vi "Send M1M3 Summary State Event.vi"(8 "error in (no error)":errorcluster, 10 "logevent_SummaryState":T1, 11 "M1M3 Support Events in":refnum<class "M1M3 Support Events.lvclass">) -> (0 "error out":errorcluster, 3 "M1M3 Support Events out":refnum<class "M1M3 Support Events.lvclass">)   [LabVIEW 2016, in "M1M3 Support Events.lvclass"]
uses:
  M1M3 Support Events.lvclass
  SALLV_m1m3/DataTypes/logevent_SummaryState.ctl
  M1M3 Support Events.lvclass/M1M3 Support Events.ctl
  SALLV_m1m3/SALLV_m1m3.lvlib
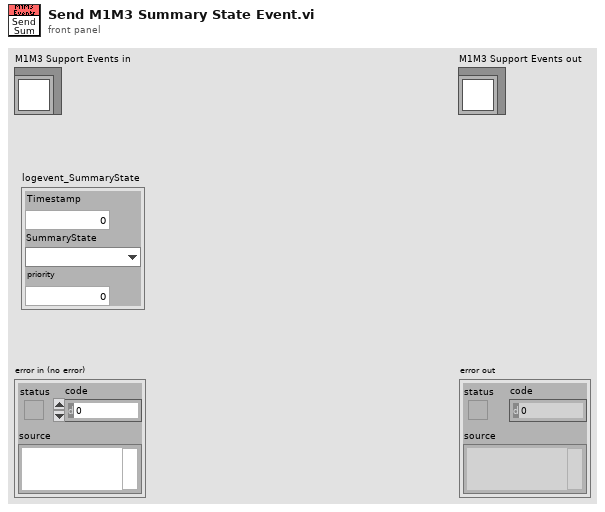
[diagram p1: front panel]
types:
  T1 = typedef "SALLV_m1m3.lvlib/logevent_SummaryState.ctl" = cluster{"Timestamp":dbl, "SummaryState":enum16{"", "SummaryState_SummaryStates_DisabledState", "SummaryState_SummaryStates_EnabledState", "SummaryState_SummaryStates_FaultState", "SummaryState_SummaryStates_OfflineState", "SummaryState_SummaryStates_StandbyState"}, "priority":i32}
  T2 = typedef "M1M3SupportEUI_TypeDefs.lvlib/M1M3 Support Events.ctl" = cluster{"Inclinometer  Data":refnum<user-event>, "IMS Data":refnum<user-event>, "SAL Connected":refnum<user-event>, "Accelerometer Data":refnum<user-event>, "OuterLoop Data":refnum<user-event>, "ErrorCode Event":refnum<user-event>, "InterlockStatus Event":refnum<user-event>, "InterlockWarning Event":refnum<user-event>, "Gyro Data":refnum<user-event>, "HP Actuator Info Event":refnum<user-event>, " FA Info Event":refnum<user-event>, "HP Monitor Info Event":refnum<user-event>, "FA Data":refnum<user-event>, "HP Actuator data":refnum<user-event>, "HP Monitor data":refnum<user-event>, "Air Supply Status Event":refnum<user-event>, "Air Supply Warning Event":refnum<user-event>, "Power Data":refnum<user-event>, "PID Data":refnum<user-event>, "PID Info Event":refnum<user-event>, "Power Status Event":refnum<user-event>, "Power Supply Status Event":refnum<user-event>, "Power Warning Event":refnum<user-event>, "Summary State Event":refnum<user-event>, "Detailed State Event":refnum<user-event>, "FA Force Warning Event":refnum<user-event>, "FA Warning Event":refnum<user-event>, "FA State Event":refnum<user-event>, "Applied AberrationForces Event":refnum<user-event>, "Applied Acceleration Forcces Event":refnum<user-event>, "Applied Azimuth Forces Event":refnum<user-event>, "Applied Active Optic Forces Event":refnum<user-event>, "Applied Balance Forces Event":refnum<user-event>, "Applied Cylinder Forces Event":refnum<user-event>, "Applied Elevation Forces Event":refnum<user-event>, "Applied Forces Event":refnum<user-event>, "Applied Offset Forces Event":refnum<user-event>, "Applied Static Forces Event":refnum<user-event>, "Applied Thermal Forces Event":refnum<user-event>, "Applied Velocity Forces Event":refnum<user-event>, "Rejected Aberration Force Event":refnum<user-event>, "Rejected Acceleration Forces Event":refnum<user-event>, "Rejected Active Optic Forces Event":refnum<user-event>, "Rejected Azimuth Forces Event":refnum<user-event>, "Rejected Balance Forces Event":refnum<user-event>, "Rejected Cylinder Forces Event":refnum<user-event>, "Rejected Elevation Forces Event":refnum<user-event>, "Rejected Forces Event":refnum<user-event>, "Rejected Offset Forces Event":refnum<user-event>, "Rejected Static Forces Event":refnum<user-event>, "Rejected Thermal Forces Event":refnum<user-event>, "Rejected Velocity Forces Event":refnum<user-event>, "Command Rejection Event":refnum<user-event>, "Setting Verions Event":refnum<user-event>, "Settings Applied Event":refnum<user-event>}
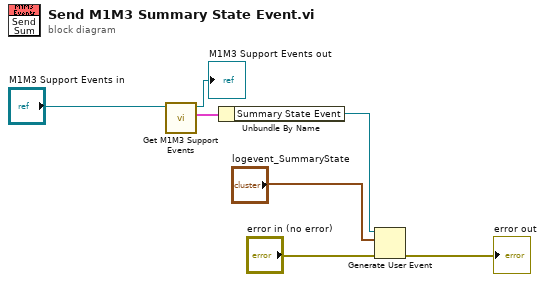
[diagram p0: block diagram]
diagram:
  n1 = call "Get M1M3 Support Events.vi"("M1M3 Support Events in"="M1M3 Support Events in") -> ("M1M3 Support Events"=w7:T2, "M1M3 Support Events out"=→"M1M3 Support Events out":refnum<class "M1M3 Support Events.lvclass">)  [unwired: 9 in]
  n2 = Unbundle By Name(w7) -> ("Summary State Event"=w6:refnum<user-event>)
  n3 = Generate User Event(user event=w6, event data cluster="logevent_SummaryState", error in="error in (no error)") -> (error out=→"error out":errorcluster)  [unwired: 1 in, 1 out]
